vi "whatMotorIs.vi"(5 "Device in":refnum<k24>) -> (1 "SerialNumber":u32, 2 "Device out":refnum<k24>)   [LabVIEW 2014]
doc: "André Romero - 2017\nandretec@ifsc.usp.br"
uses:
  C:/UserLabs/Andre/kinesis-lab13-32/kinesis-teste/Kinesis/Thorlabs.MotionControl.TCube.DCServoCLI.dll
  Kinesis/Thorlabs.MotionControl.TCube.DCServoCLI.dll
  C:/UserLabs/Andre/kinesis-lab13-32/kinesis-teste/Kinesis/Thorlabs.MotionControl.DeviceManagerCLI.dll
  Kinesis/Thorlabs.MotionControl.DeviceManagerCLI.dll
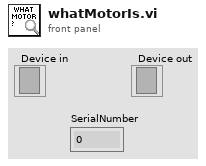
[diagram p1: front panel]
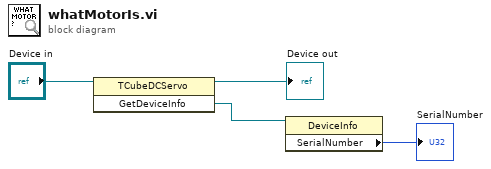
[diagram p0: block diagram]
diagram:
  n1 = invoke class="TCubeDCServo" method="GetDeviceInfo"(reference="Device in") -> (reference out=→"Device out":refnum<k24>, "GetDeviceInfo"=w2:refnum<k24>)  [unwired: 2 in, 1 out]
  n2 = property class="DeviceInfo"(reference=w2) -> ("SerialNumber"=→"SerialNumber":u32)  [unwired: 1 in, 2 out]
